vi "Read Intake Encoders.vi"   [LabVIEW 2016]
uses:
  Robot Global Data.vi
types:
  T1 = typedef "Dashboard Control Data.ctl" = cluster{"Drivetrain Settings":T2, "Intake Presets ":T5, "Shooter Presets":T6, "Vision Target Packet":T7, "Auton Presets":cluster{"Start Position":dbl}, "Drivetrain Encoder Values":T8, "Drivetrain Encoder Settings":cluster{"Left Tick Constant":dbl, "Right Tick Contant":dbl, "Reset Encoders":bool, "Center Tick Constant":dbl}, "Zero Gyro":bool, "Vision Timeout":dbl, "Pressure M":dbl, "Pressure B":dbl, "Auto Agitator":T10, "Climber Settings":T11, "LEDs":T12}
  T2 = typedef "Drivetrain Settings.ctl" = cluster{"Gyro Tolerance":dbl, "Gyro Steer PID Gains":T3, "Y Power Multiplier":dbl, "Turn Power Multiplier":dbl, "Gyro Output":dbl, "Creep Rate":dbl, "Distance Drive PID Gains":T3, "Distance Tolerance":dbl, "Distance Output":dbl, "Strafe Threshold":dbl, "Strafe Correct":bool, "Strafe Tolerance":dbl, "Translate Drive PID Gains":T3, "Strafe Output":dbl, "SC Right":dbl, "SC Left":dbl, "Use Gyro":bool, "Constant Power":bool, "Strafe Power":dbl, "Input Modifier":T4, "SCR Delay":dbl, "SCL Delay":dbl}
  T3 = typedef "PID Gains.ctl" = cluster{"proportional gain (Kc)":dbl, "integral time (Ti, min)":dbl, "derivative time (Td, min)":dbl}
  T4 = typedef "Input Modifier.ctl" = enum16{"None", "Square", "Cube"}
  T5 = typedef "Intake Presets.ctl" = cluster{"Intake Speed ":dbl, "Outake Speed":dbl, "Current Trip Delay":dbl, "Max Current":dbl, "Angle Speed":dbl, "Idle Angle":dbl, "Load Angle":dbl, "PID gains":cluster{"proportional gain (Kc)":dbl, "integral time (Ti, min)":dbl, "derivative time (Td, min)":dbl}, "Output Range":cluster{"output high":dbl, "output low":dbl}, "Angle Tolerance":dbl, "Reset Delay":dbl, "Reset Encoders?":bool, "Encoder Tick Constant ":dbl}
  T6 = typedef "Shooter Presets.ctl" = cluster{"Key Shot":cluster{"RPM ":dbl, "Hood?":bool}, "Distance Shot":cluster{"RPM":dbl, "Hood?":bool}, "RPM Tolerance":dbl, "Unstuck Delay Time ":dbl, "Initial RPM Increase":dbl, "Warmup Delay":dbl, "Faster Time":dbl, "Shooter PID Gains":cluster{"P":dbl, "I":dbl, "D":dbl, "FF":dbl, "Ramp Rate":dbl, "I Zone":dbl}, "Unstuck Trigger Power":dbl, "Trigger Power":dbl, "Unstuck RPM":dbl, "Agitator Active Power":dbl, "Agitator Idle Power":dbl, "RPM Tuning Range":dbl, "RPM M Tuning Range":dbl}
  T7 = typedef "Vision Target Packet.ctl" = cluster{"Robot Center":dbl, "Center X":dbl, "Center Y":dbl, "Angle":dbl, "Distance":dbl, "Found Target?":bool}
  T8 = typedef "Drivetrain Encoder Values.ctl" = cluster{"Left Encoder":T9, "Center Encoder":T9, "Right Encoder":T9}
  T9 = typedef "Encoder Values.ctl" = cluster{"Distance":dbl, "Speed":dbl, "Tick":dbl}
  T10 = typedef "Auto Agitator Settings.ctl" = cluster{"Enable Auto Agitation":bool, "Continuous Stir":bool, "Continuous Intake":bool, "Alternate In/Outtake":bool, "Wing Delay":dbl, "Stir Delay":dbl, "Intake Delay":dbl, "Wing On Time":dbl, "Wing Off Time":dbl, "Stir On Time":dbl, "Stir Off Time":dbl, "Intake On Time":dbl, "Intake Off Time":dbl, "Stir Power":dbl, "Intake Power":dbl, "Outtake Power":dbl, "Intake Run Time":dbl, "Outtake Run Time":dbl, "Wing$":bool, "Intake":bool, "Stirrer":bool}
  T11 = typedef "Climber Settings.ctl" = cluster{"Climber Power":dbl, "Max Current":dbl, "Avoid Current Trip?":bool}
  T12 = typedef "LED Global Data.ctl" = cluster{"Back":cluster{"Default":string, "Traction":string, "Gear Ready":string, "Break On":string, "Gear Loaded":string}, "Front":cluster{"Default":string, "Traction":string, "Gear Ready":string, "Break On":string, "Gear Loaded":string}}
  T13 = typedef "WPI_EncoderDevRef.ctl" = cluster{"DevStatus":errorcluster, "EncoderIndex":T14, "CounterIndex":T15, "DistancePerCount":dbl, "Decoding Type":T16}
  T14 = typedef "FPGA_EncoderIdx.ctl" = enum8{"Enc 0", "Enc 1", "Enc 2", "Enc 3", "Enc 4", "Enc 5", "Enc 6", "Enc 7", "Invalid"}
  T15 = typedef "FPGA_CounterCtrSystemIndex.ctl" = enum8{"Ctr 0", "Ctr 1", "Ctr 2", "Ctr 3", "Ctr 4", "Ctr 5", "Ctr 6", "Ctr 7", "Invalid"}
  T16 = typedef "WPI_EncoderType.ctl" = enum16{"1x", "2x", "4x"}
  T17 = typedef "Intake Status Cluster.ctl" = cluster{"Roller Power":dbl, "Intake Mode":T18, "Intake Auto State":T19, "Backward Tripped?":bool, "Forward Tripped?":bool, "Intake Current Trip State":T20, "Wings Open":bool, "Traction for Gear?":bool, "Current Over Max Current?":bool, "Current":dbl, "Gear Loaded":bool, "Angle Power":dbl, "Manual Angle Power":dbl, "Manual Roller Power":dbl, "Encoder Values":T9, "Tripped?":bool}
  T18 = typedef "Intake Modes.ctl" = enum16{"Manual", "Auto"}
  T19 = typedef "Intake Auto States.ctl" = enum16{"Zero", "Unload", "Load", "Idle ", "FeederStation"}
  T20 = typedef "Intake Trip States.ctl" = enum16{"Normal", "Backward Tripped", "Forward Tripped"}
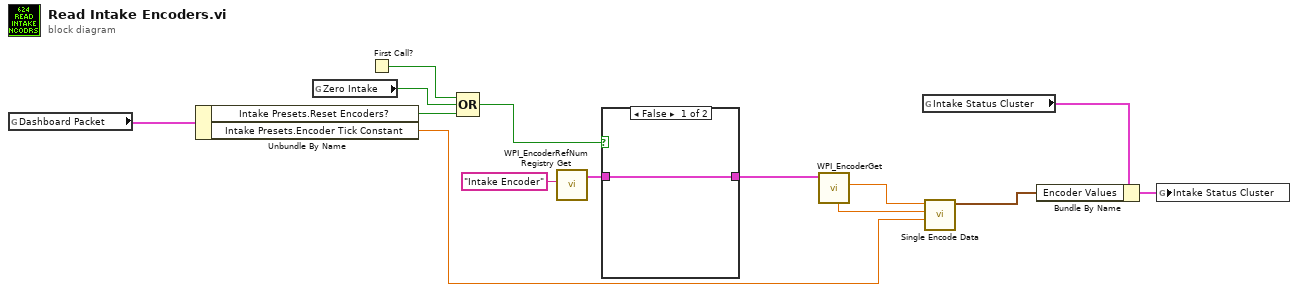
[diagram p0: block diagram]
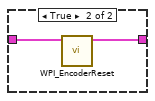
[diagram p2: hidden frame]
diagram:
  n1 = global read "Robot Global Data.vi" "Dashboard Packet"() -> (w9:T1)
  n2 = Unbundle By Name(w9) -> ("Intake Presets.Reset Encoders?"=w8:bool, "Intake Presets.Encoder Tick Constant"=w4:dbl)
  n3 = global read "Robot Global Data.vi" "Zero Intake"() -> (w7:bool)
  n4 = First Call?() -> (First Call?: T/F=w6:bool)
  n5 = Compound Arithmetic op=OR(w6, w7, w8) -> (w5:bool)
  n6 = call <vilib>:"WPI_EncoderRefNum Registry Get.vi"("refnum name"="Intake Encoder") -> ("EncoderDevRef"=w11:T13)  [unwired: 9 in, 1 out]
  n7 = case shown="False" w5 {
    tunnel: w11 -> [w15 w17]
    tunnel: [w15 w16] -> w10
    frame False {
    }
    frame True {
      n8 = call <vilib>:"WPI_EncoderReset.vi"("EncoderDevRef"=w17) -> ("EncoderDevRef"=w16:T13)  [unwired: 9 in, 1 out]
    }
  }
  n9 = call <vilib>:"WPI_EncoderGet.vi"("EncoderDevRef"=w10) -> ("Distance"=w14:dbl, "Rate"=w13:dbl)  [unwired: 5 in, 4 out]
  n10 = global read "Robot Global Data.vi" "Intake Status Cluster"() -> (w3:T17)
  n11 = call "Single Encode Data.vi"("Tick Constant"=w4, "Rate"=w13, "Distance"=w14) -> ("Encoder Values"=w1:T9)  [unwired: 8 in]
  n12 = Bundle By Name(cluster=w3, "Encoder Values"=w1) -> (w2:T17)
  n13 = global write "Robot Global Data.vi" "Intake Status Cluster"(w2) -> ()
